vi "Manual with LIDAR localisation - testing (with obst avd).vi"() -> ()   [LabVIEW 2017]
uses:
  <instrlib>/Hokuyo URG Series/Hokuyo URG Series.lvlib
  <vilib>/ptbypt/NI_PtbyPt.lvlib
  <instrlib>/Hokuyo URG Series/Public/Initialize-cRIO-USB.vi
panel:
  out "Motor C out":dbl(graph)
  out "Motor B out":dbl(graph)
  out "Motor A out":dbl(graph)
  out "dt":u32(graph)
  out "dt (localisation)":u32
  out "dx dy":cluster{"x":dbl, "y":dbl}
  out "xy est":cluster{"x":dbl, "y":dbl} {"y" format="%#.6f"; "x" format="%#.6f"}
  out "Counter C0":i32
  out "Counter B0":i32
  out "Counter A0":i32
  out "LIDAR Angle":dbl
  out "No lines big enough":bool
  in  "Ignore values less than []":dbl=180.0 format="%#_13g"
  in  "Obstacle detect distance":dbl=220.0
  out "Angle to move out":dbl
  out "desired movement angle":dbl
  out "Obstacle angle":i32
  out "min dist":dbl
  out "Obstacle detected":bool
  out "Gyro calibration finished":bool
  in  "Desired orientation":dbl
  in  "Orientation for max rotation":dbl=30.0
  in  "Localisation period":i64=100
  out "LOST":bool
  out "dy":dbl
  out "dx":dbl
  in  "Delay (s)":dbl
  out "Remaining delay":dbl
  out "y ref":dbl
  out "y":dbl
  out "x ref":dbl
  out "x":dbl
  in  "Min orientation for rotation":dbl=5.0
  in  "Rot min abs spd":dbl=0.5
  in  "Motor Stop (esc)":bool
  out "Ann Nee loc\nCurrent position":cluster{"X":dbl, "Y":dbl}
  out "orientation angle":dbl format="%0.10f"
  out "xgTest":u8
  in  "Initial position":cluster{"X":dbl, "Y":dbl}={"X"=750.0, "Y"=3700.0}
  in  "Right":bool
  in  "Left":bool
  in  "Down":bool
  in  "Up":bool
  in  "Fast period":i64=10
  in  "Protocol":u32(ring)=2 items=["Convert to Latest", "SCIP 1.1", "SCIP 2.0"]
  in  "ID Query?":bool=TRUE
  in  "Checksum":bool
  in  "Stop":bool
  out "XY Graph 6m max":cluster{"Y":dbl[], "Y":dbl[]}[](graph)
  in  "Rot spd multiplier":dbl=2.0
  in  "error in":errorcluster
  in  "Trans spd multiplier":dbl=2.0
  in  "PID gains":T1={"proportional gain (Kc)"=0.015, "integral time (Ti, min)"=0.003, "derivative time (Td, min)"=0.0} {"derivative time (Td, min)" format="%.6f"; "integral time (Ti, min)" format="%.6f"; "proportional gain (Kc)" format="%.6f"}
  # "P:  Higher the number, higher the abrupt change\nI: Higher the number, the less it tries to overshoot"
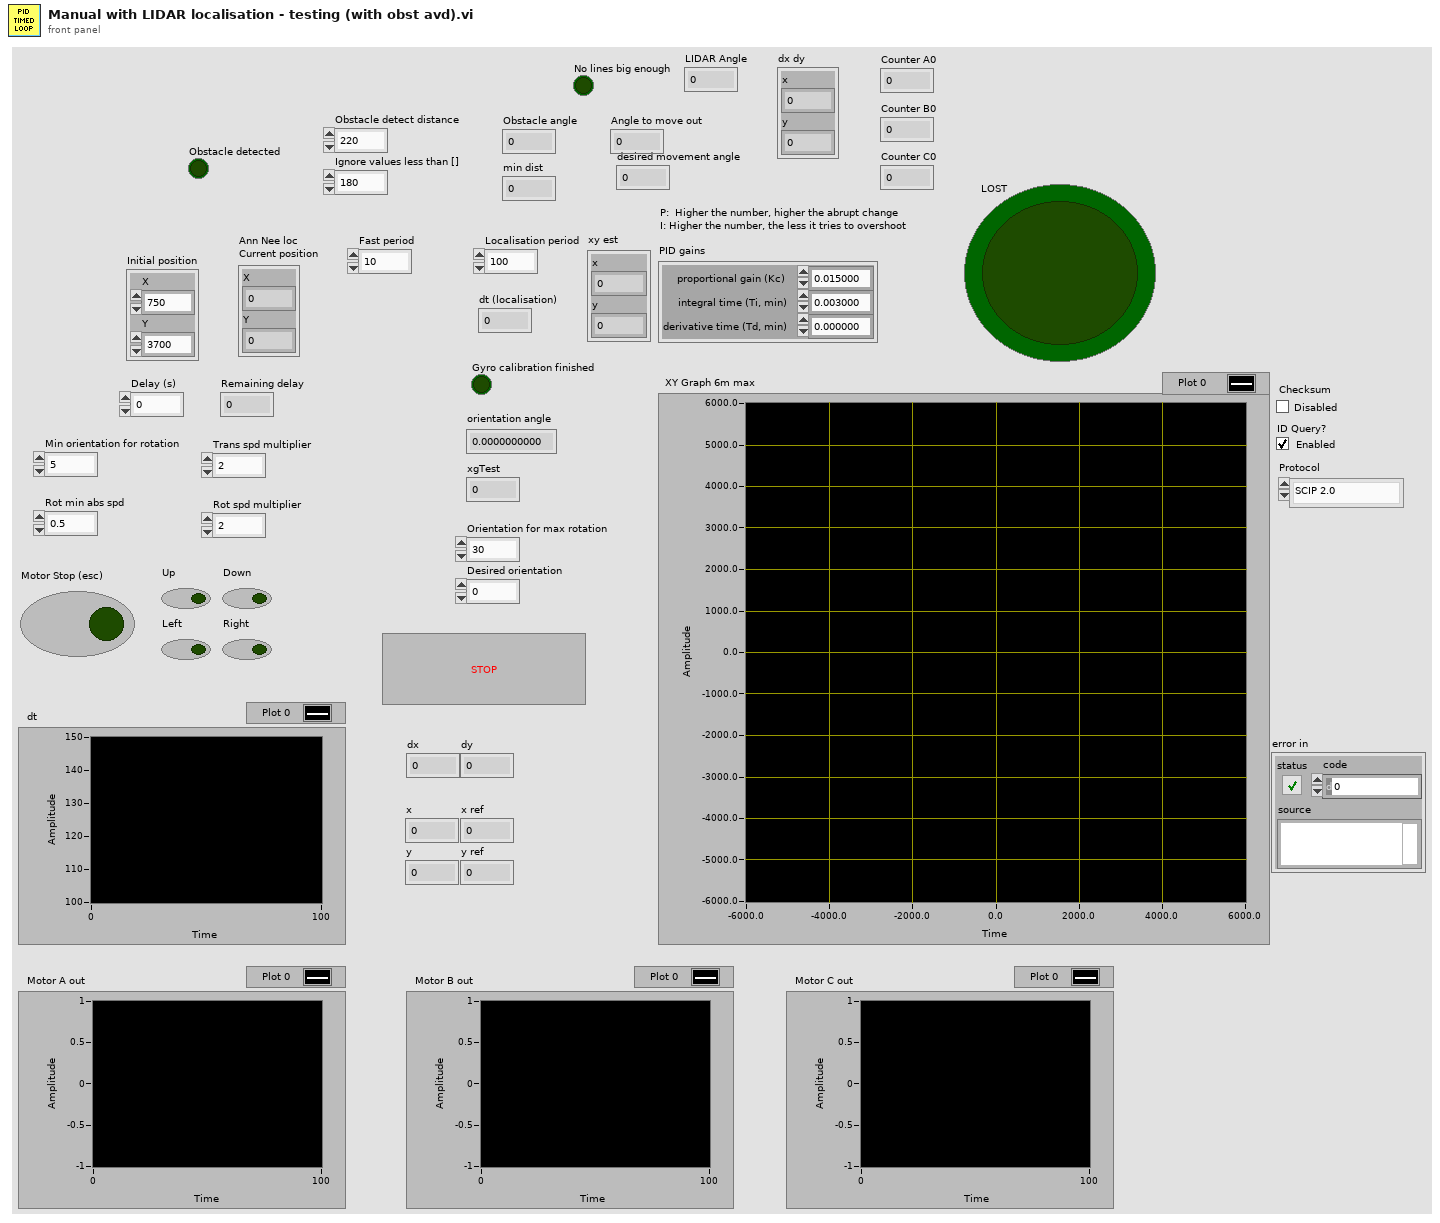
[diagram p1: front panel]
types:
  T1 = cluster{"proportional gain (Kc)":dbl, "integral time (Ti, min)":dbl, "derivative time (Td, min)":dbl}
  T2 = enum16{"Stop / None", "Forward", "Backward", "Left", "Right", "Manual"}
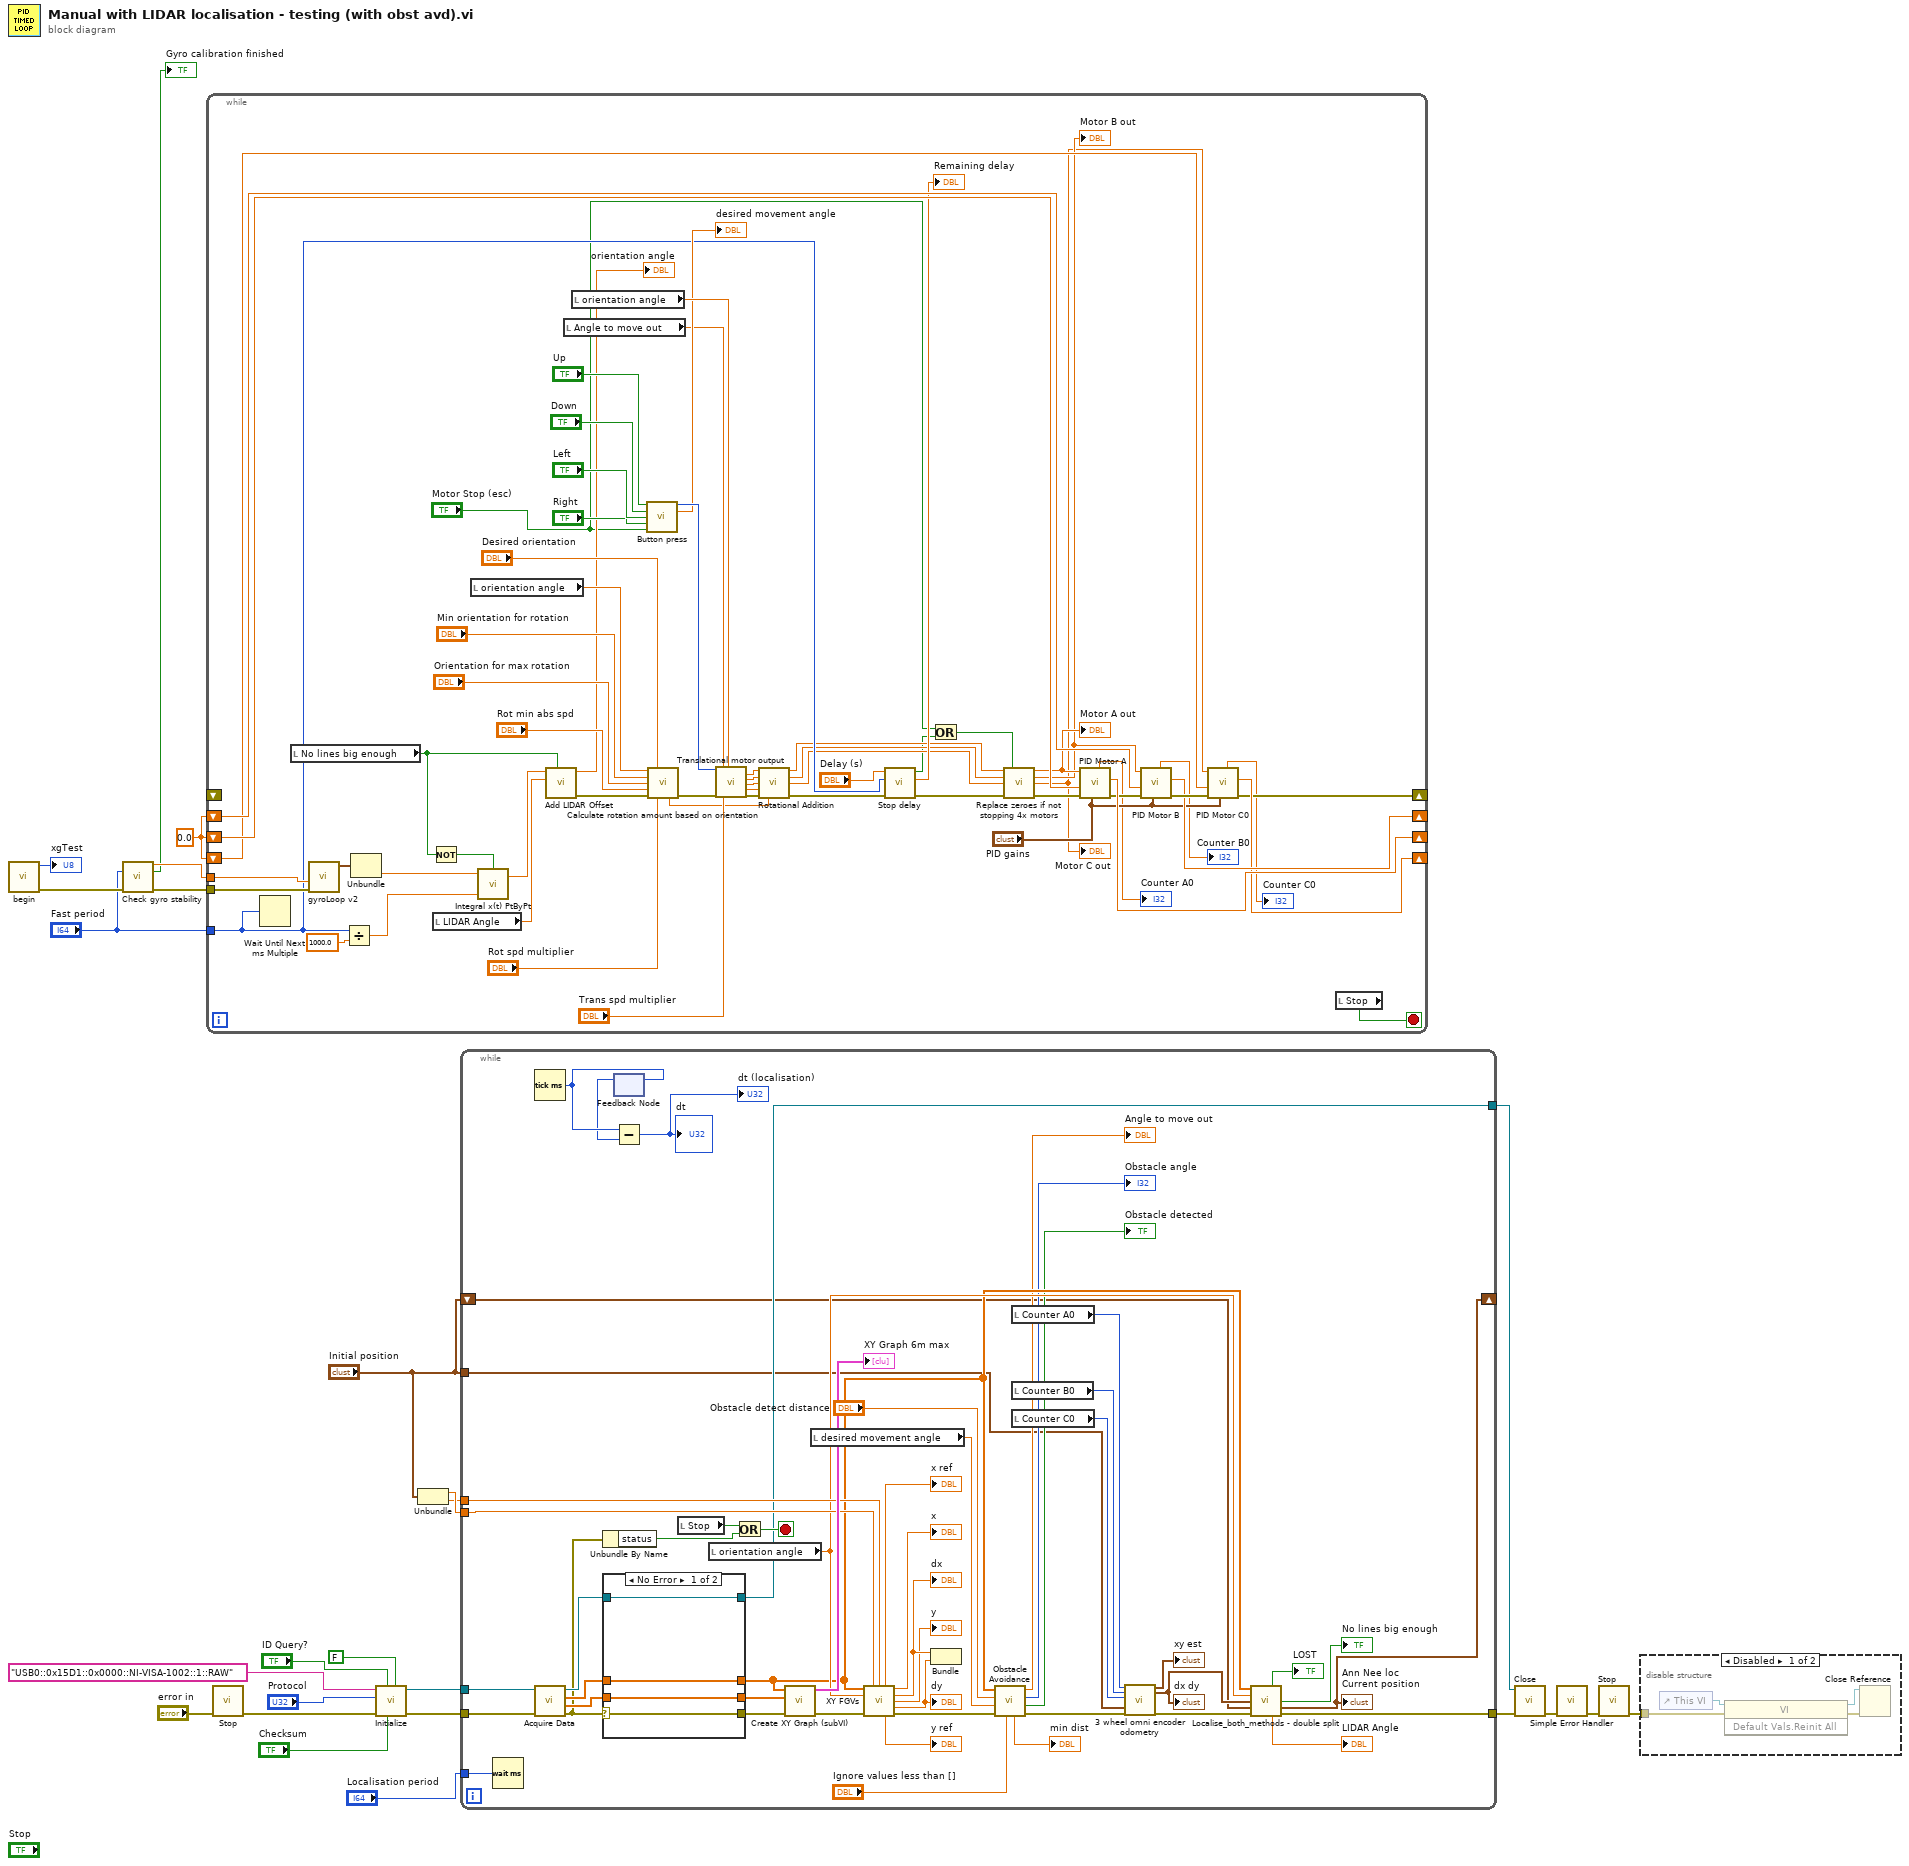
[diagram p0: block diagram]
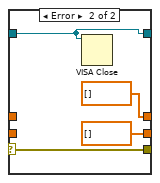
[diagram p2: hidden frame]
diagram:
  w20 = 0.0 ("output")
  n1 = call "begin.vi"() -> ("Error out"=w9:errorcluster, "xgTest"=→"xgTest":u8)  [unwired: 10 in]
  n2 = call "Check gyro stability.vi"("Period"="Fast period", "error in (no error)"=w9) -> ("gz offset"=w7:dbl, "Gyro calibration finished"=→"Gyro calibration finished":bool, "error out"=w8:errorcluster)  [unwired: 11 in]
  n3 = while {
    shift-right: [w87] -> _
    shift-left: w20 -> [w88]
    shift-right: [w82] -> _
    shift-left: w20 -> [w81]
    shift-right: [w84] -> _
    shift-left: w20 -> [w83]
    shift-right: [w40] -> _
    shift-left: _ -> [_]
    tunnel: w8 -> [w55]
    tunnel: w7 -> [w54]
    tunnel: "Fast period" -> [w47]
    stop <- w56 stop-if-true
    n4 = Wait Until Next ms Multiple(millisecond multiple=w47) -> ()  [unwired: 1 out]
    n5 = local read "No lines big enough"() -> (w41:bool)
    n6 = call "gyroLoop v2.vi"("Error in"=w55, "gzOffset"=w54) -> ("Velocities Graph"=w57:cluster{dbl, dbl, dbl})  [unwired: 7 in, 2 out]
    n7 = Divide(x=w47, y=1000.0) -> (x/y=w48:dbl)
    n8 = Unbundle(w57) -> (w58:dbl)  [unwired: 2 out]
    n9 = Not(x=w41) -> (.not. x?=w42:bool)
    n10 = local read "LIDAR Angle"() -> (w43:dbl)
    n11 = local read "orientation angle"() -> (w60:dbl)
    n12 = call <vilib>:"Integral x(t) PtByPt.vi"("initialize"=w42, "dt"=w48, "x"=w58) -> ("integral x(t)"=w46:dbl)  [unwired: 1 in, 1 out]
    n13 = call "Add LIDAR Offset.vi"("Lost?"=w41, "LIDAR Angle"=w43, "New gyro reading"=w46) -> ("error out"=w44:errorcluster, "new angle"=→"orientation angle":dbl)  [unwired: 7 in]
    n14 = local read "Angle to move out"() -> (w49:dbl)
    n15 = local read "orientation angle"() -> (w66:dbl)
    n16 = call "Button press.vi"("Up"="Up", "Down"="Down", "Left"="Left", "Right"="Right", "Stop"="Motor Stop (esc)") -> ("Command"=w73:T2, "angle"=→"desired movement angle":dbl)  [unwired: 9 in]
    n17 = call "Calculate rotation amount based on orientation.vi"("Orientation"=w60, "Desired orientation"="Desired orientation", "Min orientation for rotation"="Min orientation for rotation", "Orientation for max rotation"="Orientation for max rotation", "Rot min abs spd"="Rot min abs spd", "error in"=w44, "Rot spd multiplier"="Rot spd multiplier") -> ("Rot spd out"=w67:dbl, "error out"=w50:errorcluster)  [unwired: 5 in, 2 out]
    n18 = call "Translational motor output.vi"("Command"=w73, "error in"=w50, "manual input angle"=w49, "Trans spd multiplier"="Trans spd multiplier", "Orientation"=w66) -> ("motor 1 out"=w75:dbl, "motor 2 out"=w76:dbl, "motor 3 out"=w77:dbl, "motor 4 out"=w78:dbl, "error out"=w79:errorcluster)  [unwired: 10 in]
    n19 = call "Rotational Addition.vi"("Motor 1 in"=w75, "Motor 2 in"=w76, "Motor 3 in"=w77, "Motor 4 in"=w78, "error in"=w79, "Rot spd multiplier"=w67) -> ("Motor 1 out"=w34:dbl, "Motor 2 out"=w33:dbl, "Motor 3 out"=w32:dbl, "error out"=w65:errorcluster)  [unwired: 5 in, 1 out]
    n20 = call "Stop delay.vi"("error in (no error)"=w65, "Period (ms)"=w47, "Delay (s)"="Delay (s)") -> ("error out"=w36:errorcluster, "Remaining delay"=→"Remaining delay":dbl, "Stop?"=w30:bool)  [unwired: 6 in]
    n21 = Or(x="Motor Stop (esc)", y=w30) -> (x .or. y?=w29:bool)
    n22 = call "Replace zeroes if not stopping 4x motors.vi"("Motor 1 in"=w34, "Stop?"=w29, "Motor 2 in"=w33, "Motor 3 in"=w32, "error in (no error)"=w36) -> ("Motor 1 out"=w28:dbl, "Motor 2 out"=w27:dbl, "Motor 3 out"=w26:dbl, "error out"=w35:errorcluster)  [unwired: 6 in, 1 out]
    "Motor A out" <- w28
    "Motor B out" <- w27
    "Motor C out" <- w26
    n23 = call "PID Motor A.vi"("PID gains"="PID gains", "error in (no error)"=w35, "input"=w88, "Setpoint A0"=w28) -> ("error out"=w86:errorcluster, "output"=w87:dbl, "Counter A0"=→"Counter A0":dbl)  [unwired: 2 in, 3 out]
    n24 = call "PID Motor B.vi"("PID gains"="PID gains", "error in (no error)"=w86, "input"=w83, "Setpoint B0"=w27) -> ("error out"=w85:errorcluster, "output"=w84:dbl, "Counter B0"=→"Counter B0":dbl)  [unwired: 2 in, 3 out]
    n25 = call "PID Motor C0.vi"("PID gains"="PID gains", "error in (no error)"=w85, "input"=w81, "Setpoint C0"=w26) -> ("error out"=w40:errorcluster, "output"=w82:dbl, "Counter C0"=→"Counter C0":dbl)  [unwired: 2 in, 3 out]
    n26 = local read "Stop"() -> (w56:bool)
  }
  n27 = call "Stop.vi"("error in (no error)"="error in") -> ("OG error out"=w2:errorcluster)  [unwired: 9 in, 1 out]
  n28 = call-poly <instrlib>:"Initialize.vi"("Reset? (F: No)"=FALSE ("Reset Instrument (Disabled)"), "Checksum (Disabled)"="Checksum", "ID Query? (Enabled)"="ID Query?", "error in (no error)"=w2, "Protocol (2: SCIP 2.0)"="Protocol", "VISA resource name"="USB0::0x15D1::0x0000::NI-VISA-1002::1::RAW") -> ("error out"=w16:errorcluster, "VISA resource name out"=w15:refnum<visa-resource-name>)  [unwired: 4 in]
  n29 = Unbundle("Initial position") -> ("X"=w18:dbl, "Y"=w17:dbl)
  n30 = while {
    tunnel: w18 -> [w123]
    tunnel: w17 -> [w122]
    shift-right: [w106] -> _
    shift-left: "Initial position" -> [w96]
    tunnel: w16 -> [w120]
    tunnel: w15 -> [w119]
    tunnel: [w105] -> w11
    tunnel: [w118] -> w10
    tunnel: "Localisation period" -> [w104]
    tunnel: "Initial position" -> [w94]
    stop <- w121 stop-if-true
    n31 = Wait (ms)(milliseconds to wait=w104) -> ()  [unwired: 1 out]
    n32 = Tick Count (ms)() -> (millisecond timer value=w91:u32)
    n33 = call <instrlib>:"Acquire Data.vi"("error in (no error)"=w120, "VISA resource name"=w119) -> ("error out"=w127:errorcluster, "Direction"=w128:dbl[], "Magnitude"=w130:dbl[], "VISA resource name out"=w129:refnum<visa-resource-name>)  [unwired: 6 in]
    n34 = Unbundle By Name(w127) -> ("status"=w92:bool)
    n35 = case shown="No Error" w127 {
      selector: w127 -> [w139 w146]
      tunnel: [w139 w146] -> w124
      tunnel: w129 -> [w142 w145]
      tunnel: [w142 w145] -> w118
      tunnel: w130 -> [w141 _]
      tunnel: w128 -> [w140 _]
      tunnel: [w141 dbl[] [] ("Magnitude")] -> w115
      tunnel: [w140 dbl[] [] ("Direction")] -> w125
      frame No Error {
      }
      frame Error {
        n36 = VISA Close(VISA resource name=w145) -> ()  [unwired: 1 in, 1 out]
      }
    }
    n37 = feedback-in #1(w91) -> ()
    n38 = feedback #1() -> (w90:u32)  [unwired: 1 in]
    n39 = Subtract(x=w91, y=w90) -> (x-y=→"dt (localisation)" →"dt":u32)
    n40 = local read "Stop"() -> (w93:bool)
    n41 = local read "orientation angle"() -> (w117:dbl)
    n42 = Or(x=w93, y=w92) -> (x .or. y?=w121:bool)
    n43 = call "Create XY Graph (subVI).vi"("error in"=w124, "Direction"=w125, "Magnitude"=w115) -> ("error out"=w131:errorcluster, "XY Graph"=→"XY Graph 6m max":cluster{"Y":dbl[], "Y":dbl[]}[])  [unwired: 6 in, 1 out]
    n44 = local read "desired movement angle"() -> (w116:dbl)
    n45 = call "XY FGVs.vi"("LIDAR Mag"=w115, "x init"=w123, "y init"=w122, "Orientation\n(anticlockwise)"=w117, "error in (no error)"=w131) -> ("x ref"=→"x ref":dbl, "x"=→"x":dbl, "dx"=w136:dbl, "y"=→"y":dbl, "dy"=w137:dbl, "y ref"=→"y ref":dbl, "error out"=w109:errorcluster)  [unwired: 4 in]
    "dx" <- w136
    "dy" <- w137
    n46 = Bundle("dx"=w136, "dy"=w137) -> ()  [unwired: 1 in, 1 out]
    n47 = call "Obstacle Avoidance.vi"("Ignore values less than []"="Ignore values less than []", "error in (no error)"=w109, "Desired angle to move"=w116, "Obstacle detect distance"="Obstacle detect distance", "LIDAR"=w115) -> ("error out"=w102:errorcluster, "Obstacle detected"=→"Obstacle detected":bool, "Obstacle angle"=→"Obstacle angle":i32, "Angle to move out"=→"Angle to move out":dbl, "min dist"=→"min dist":dbl)  [unwired: 2 in]
    n48 = local read "Counter A0"() -> (w99:i32)
    n49 = local read "Counter B0"() -> (w98:i32)
    n50 = local read "Counter C0"() -> (w97:i32)
    n51 = call "3 wheel omni encoder odometry.vi"("Motor 1 Encoder"=w99, "Motor 2 Encoder"=w98, "Motor 3 Encoder"=w97, "Initial position"=w94, "error in (no error)"=w102) -> ("xy est"=→"xy est":cluster{"x":dbl, "y":dbl}, "dx dy"=w100:cluster{"x":dbl, "y":dbl}, "error out"=w101:errorcluster)  [unwired: 10 in, 2 out]
    "dx dy" <- w100
    n52 = call "Localise_both_methods - double split.vi"("LIDAR"=w115, "EIstimated angle (degrees)"=w117, "Offset From Encoders"=w100, "Previous Position"=w96, "error in (no error)"=w101) -> ("LOST"=→"LOST":bool, "No lines big enough"=→"No lines big enough":bool, "Localised position"=w106:cluster{"X":dbl, "Y":dbl}, "Corrected Angle"=→"LIDAR Angle":dbl, "error out"=w105:errorcluster)  [unwired: 3 in, 3 out]
    "Ann Nee loc\nCurrent position" <- w106
  }
  n53 = call <instrlib>:"Close.vi"("error in (no error)"=w11, "VISA resource name"=w10) -> ("error out"=w13:errorcluster)  [unwired: 9 in]
  n54 = call <vilib>:"Simple Error Handler.vi"("error in (no error)"=w13) -> ("error out"=w12:errorcluster)  [unwired: 4 in, 4 out]
  n55 = call "Stop.vi"("error in (no error)"=w12) -> ("OG error out"=w14:errorcluster)  [unwired: 9 in, 1 out]
  n56 = disable-structure shown="Disabled" {
    disable-tunnel: w14 -> [w147 _]
    frame Disabled {
      n57 = control-ref of="This VI"() -> (w150:refnum<vi>)
      n58 = invoke class="VI" method="Default Vals.Reinit All"(reference=w150, error in=w147) -> (reference out=w149:refnum<vi>, error out=w148:errorcluster)  [unwired: 1 in, 1 out]
      n59 = Close Reference(reference=w149, error in (no error)=w148) -> ()  [unwired: 1 out]
    }
    frame Enabled {
    }
  }
